vi "Generate.vi"(0 "reference in":refnum<class "Python.lvclass">, 1 "Path":path, 3 "Classes":T1[](array[typedef]), 5 "error in (no error)":errorcluster) -> (14 "reference out":refnum<class "Python.lvclass">, 19 "error out":errorcluster)   [LabVIEW 2018, in "Python.lvclass"]
uses:
  Python.lvclass
  Executer_class/typedefs/ClassDescription.ctl
  Executer_class/typedefs/MethodDescription.ctl
  Executer_class/Executer.lvclass
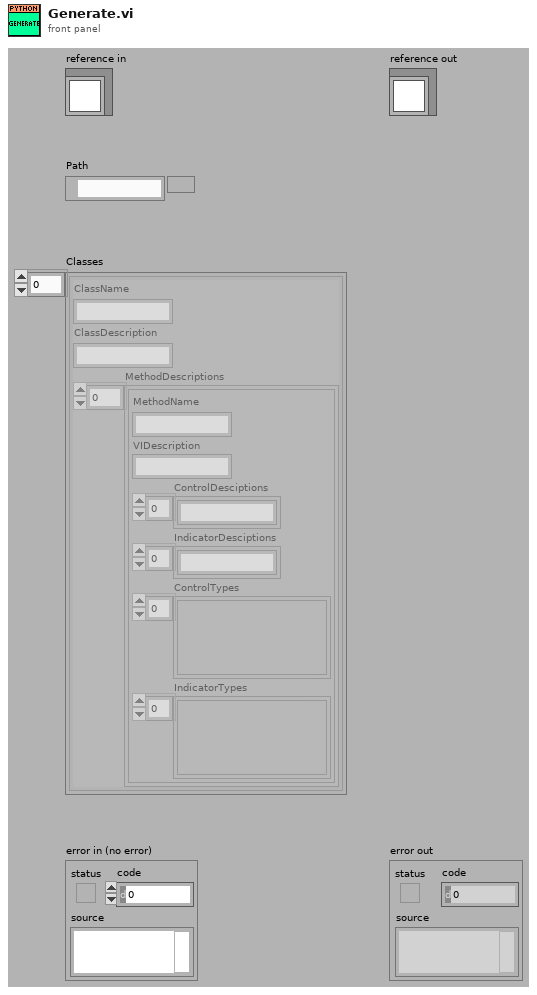
[diagram p1: front panel]
types:
  T1 = typedef "Executer.lvclass/ClassDescription.ctl" = cluster{"ClassName":string, "ClassDescription":string, "MethodDescriptions":T2[]}
  T2 = typedef "Executer.lvclass/MethodDescription.ctl" = cluster{"MethodName":string, "VIDescription":string, "ControlDesciptions":string[], "IndicatorDesciptions":string[], "ControlTypes":variant[], "IndicatorTypes":variant[]}
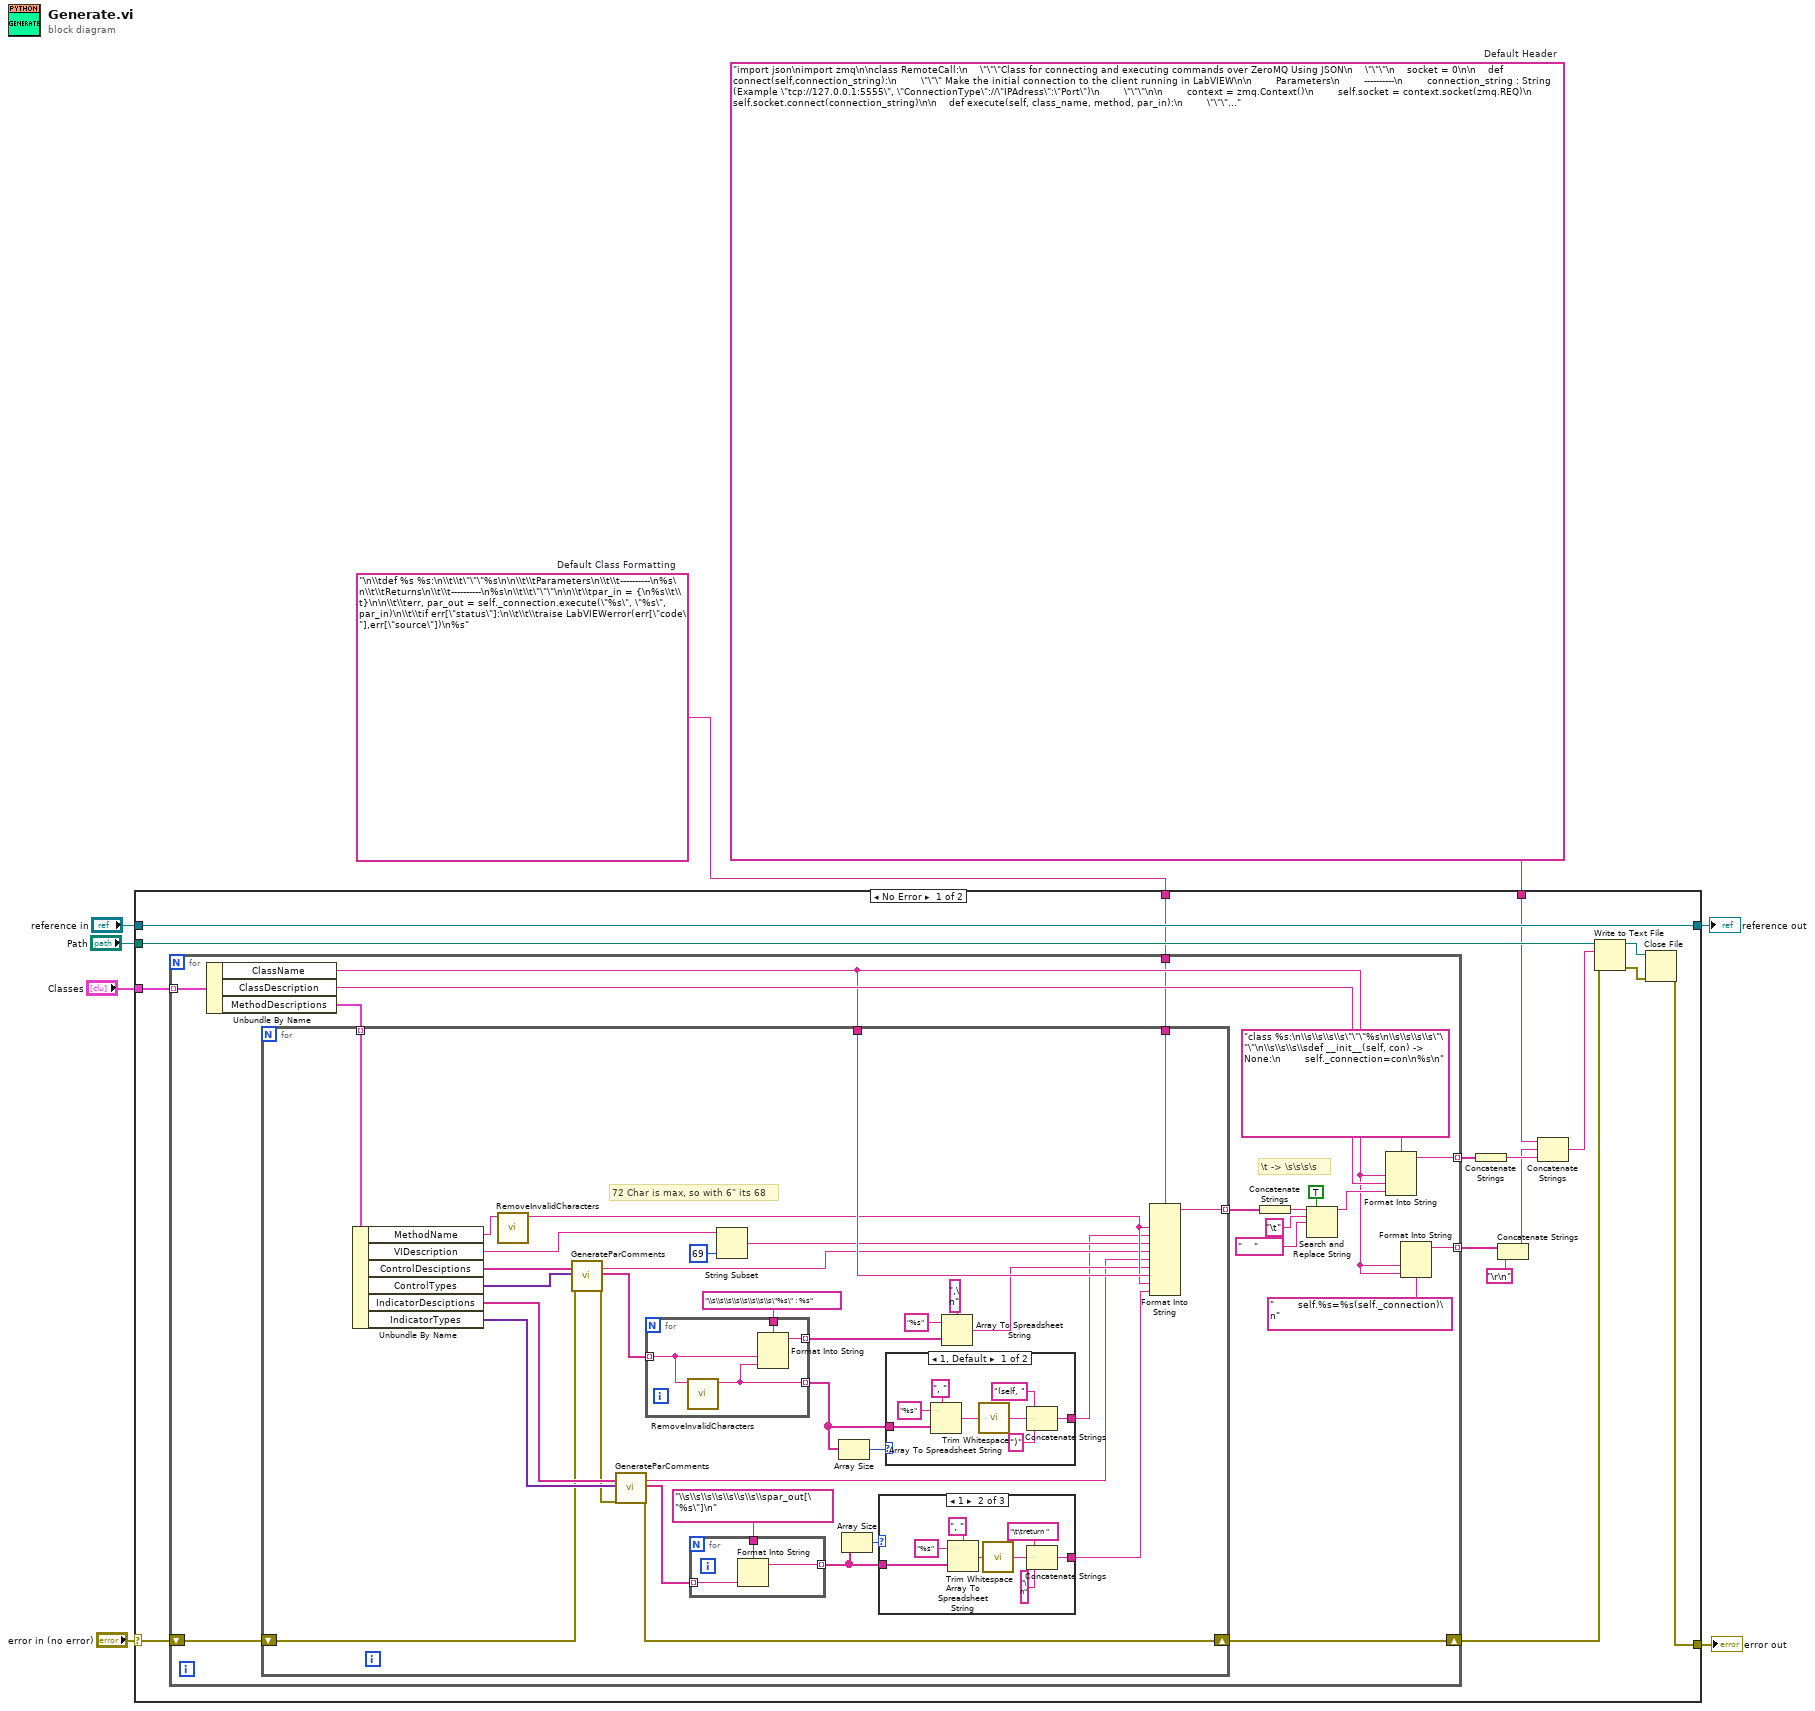
[diagram p0: block diagram]
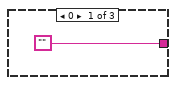
[diagram p2: hidden frame]
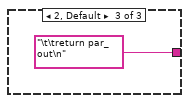
[diagram p3: hidden frame]
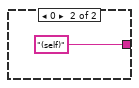
[diagram p4: hidden frame]
diagram:
  w1 = "\n\\tdef %s %s:\n\\t\\t\"\"\"%s\n\n\\t\\tParameters\n\\t\\t----------\n%s\n\\t\\tReturns\n\\t\\t----------\n%s\n\\t\\t\"\"\"\n\n\\t\\tpar_in = {\n%s\\t\\t}\n\n\\t\\terr, par_out = self._connection.execute(\"%s\", \"%s\", par_in)\n\\t\\tif err[\"status\"]:\n\\t\\t\\traise LabVIEWerror(err[\"code\"],err[\"source\"])\n%s"  # Default Class Formatting
  w2 = "import json\nimport zmq\n\nclass RemoteCall:\n    \"\"\"Class for connecting and executing commands over ZeroMQ Using JSON\n    \"\"\"\n    socket = 0\n\n    def connect(self,connection_string):\n        \"\"\" Make the initial connection to the client running in LabVIEW\n\n        Parameters\n        ----------\n        connection_string : String (Example \"tcp://127.0.0.1:5555\", \"ConnectionType\"://\"IPAdress\":\"Port\")\n        \"\"\"\n\n        context = zmq.Context()\n        self.socket = context.socket(zmq.REQ)\n        self.socket.connect(connection_string)\n\n    def execute(self, class_name, method, par_in):\n        \"\"\" Execute the Method by serializing inputs sending it over, and deserializing the result\n        \"\"\"\n        data_2_send = \"{ \\\"Command\\\":\\\"Execute\\\" }\\x17{\\\"ClassLabel\\\":\\\"%s\\\",\\\"Method\\\":\\\"%s\\\"}\\x17%s\" % (class_name, method, json.dumps({\"In\": par_in}))\n        self.socket.send_string (data_2_send)\n        message = self.socket.recv()\n        parts = message.split(chr(0x17).encode())\n        return json.loads(parts[1]), json.loads(parts[0])\n\nclass LabVIEWerror(Exception):\n    \"\"\"Base class for all LabVIEW errors\n\n    Attributes\n    ----------\n    code: error code for testing which error happend\n    source: source of the error\n    \"\"\"\n    def __init__(self, *args: object) -> None:\n        self.code = self.args[0]\n        self.source = self.args[1]\n        super().__init__(*args)\n\n    def __str__(self) -> str:\n        return f\"LabVIEW Error with code: {self.code} source: {self.source}\"\n\nclass LabviewControl:\n    \"\"\" Class for calling all labview function with connection embedded\n    \"\"\"\n\n    def __init__(self,connection_string) -> None:\n        self._connection=RemoteCall()\n        self._connection.connect(connection_string)\n"  # Default Header
  n1 = case shown="No Error" "error in (no error)" {
    selector: "error in (no error)" -> [w16 w101]
    tunnel: [w19 w101] -> w7
    tunnel: [w17 w100] -> w5
    tunnel: "reference in" -> [w17 w100]
    tunnel: "Classes" -> [w15 _]
    tunnel: "Path" -> [w14 _]
    tunnel: w2 -> [w12 _]
    tunnel: w1 -> [w9 _]
    frame No Error {
      n2 = for {
        tunnel: [w41] -> w24 mode=indexing
        tunnel: w15 -> [w31] mode=indexing
        shift-right: [w33] -> w18
        shift-left: w16 -> [w32]
        tunnel: [w26] -> w13 mode=indexing
        tunnel: w9 -> [w25]
        # "\\t -> \\s\\s\\s\\s"
        n3 = Unbundle By Name(w31) -> ("ClassName"=w27:string, "ClassDescription"=w30:string, "MethodDescriptions"=w29:T2[])
        n4 = for {
          tunnel: [w73] -> w40 mode=indexing
          tunnel: w27 -> [w72]
          shift-right: [w47] -> w33
          shift-left: w32 -> [w49]
          tunnel: w29 -> [w46] mode=indexing
          tunnel: w25 -> [w44]
          # "72 Char is max, so with 6\" its 68"
          n5 = Unbundle By Name(w46) -> ("MethodName"=w45:string, "VIDescription"=w61:string, "ControlDesciptions"=w60:string[], "ControlTypes"=w59:variant[], "IndicatorDesciptions"=w50:string[], "IndicatorTypes"=w51:variant[])
          n6 = call "RemoveInvalidCharacters.vi"("string in"=w45) -> ("string out"=w71:string)  [unwired: 10 in]
          n7 = call "GenerateParComments.vi"("Desciptions"=w60, "Types"=w59, "error in (no error)"=w49) -> ("DescriptionString"=w58:string, "Names"=w56:string[], "error out"=w48:errorcluster)  [unwired: 14 in]
          n8 = call "GenerateParComments.vi"("Desciptions"=w50, "Types"=w51, "error in (no error)"=w48) -> ("DescriptionString"=w57:string, "Names"=w55:string[], "error out"=w47:errorcluster)  [unwired: 14 in]
          n9 = for {
            tunnel: [w90] -> w65 mode=indexing
            tunnel: [w89] -> w53 mode=indexing
            tunnel: w56 -> [w88] mode=indexing
            tunnel: "\\s\\s\\s\\s\\s\\s\\s\\s\"%s\" : %s" ("string") -> [w87]
            n10 = call "RemoveInvalidCharacters.vi"("string in"=w88) -> ("string out"=w89:string)  [unwired: 10 in]
            n11 = Format Into String(format string=w87, w88, w89) -> (resulting string=w90:string)  [unwired: 2 in, 1 out]
          }
          n12 = for {
            tunnel: [w86] -> w66 mode=indexing
            tunnel: w55 -> [w85] mode=indexing
            tunnel: "\\s\\s\\s\\s\\s\\s\\s\\spar_out[\"%s\"]\n" ("string") -> [w84]
            n13 = Format Into String(format string=w84, w85) -> (resulting string=w86:string)  [unwired: 2 in, 1 out]
          }
          n14 = String Subset(string=w61, length (rest)=69 ("length (rest)")) -> (substring=w70:string)  [unwired: 1 in]
          n15 = Array Size(array=w53) -> (size(s)=w52:i32)
          n16 = Array Size(array=w66) -> (size(s)=w68:i32)
          n17 = case shown="1" w68 {
            tunnel: ["" w82 "\t\treturn par_out\n" ("string")] -> w67
            tunnel: w66 -> [_ w76 _]
            frame 0 {
            }
            frame 1 {
              n18 = Array To Spreadsheet String(delimiter (Tab)=", ", array=w76, 3:"%s" ("format string")) -> (spreadsheet string=w77:string)
              n19 = call <vilib>:"Trim Whitespace.vi"("string"=w77) -> ("trimmed string"=w75:string)  [unwired: 1 in]
              n20 = Concatenate Strings("\t\treturn " ("string"), w75, "\n" ("delimiter (Tab)")) -> (w82:string)
            }
            frame 2, Default {
            }
          }
          n21 = case shown="1, Default" w52 {
            tunnel: [w91 "(self)" ("string")] -> w54
            tunnel: w53 -> [w92 _]
            frame 1, Default {
              n22 = Array To Spreadsheet String(delimiter (Tab)=", ", array=w92, 3:"%s" ("format string")) -> (spreadsheet string=w95:string)
              n23 = call <vilib>:"Trim Whitespace.vi"("string"=w95) -> ("trimmed string"=w97:string)  [unwired: 1 in]
              n24 = Concatenate Strings("(self, " ("string"), w97, ")" ("string")) -> (w91:string)
            }
            frame 0 {
            }
          }
          n25 = Array To Spreadsheet String(delimiter (Tab)=",\n", array=w65, 3:"%s" ("format string")) -> (spreadsheet string=w62:string)
          n26 = Format Into String(format string=w44, w71, w54, w70, w58, w57, w62, w72, w71, w67) -> (resulting string=w73:string)  [unwired: 2 in, 1 out]
        }
        n27 = Concatenate Strings(w40) -> (w39:string)
        n28 = Search and Replace String(replace all?=TRUE ("replace all? (F)"), input string=w39, search string="\t", replace string="    " ("search string")) -> (result string=w34:string)  [unwired: 4 in, 3 out]
        n29 = Format Into String(format string="class %s:\n\\s\\s\\s\\s\"\"\"%s\n\\s\\s\\s\\s\"\"\"\n\\s\\s\\s\\sdef __init__(self, con) -> None:\n        self._connection=con\n%s\n", w27, w30, w34) -> (resulting string=w41:string)  [unwired: 2 in, 1 out]
        n30 = Format Into String(format string="        self.%s=%s(self._connection)\n", w27, w27) -> (resulting string=w26:string)  [unwired: 2 in, 1 out]
      }
      n31 = Concatenate Strings(w24) -> (w23:string)
      n32 = Concatenate Strings(w13, "\r\n") -> (w11:string)
      n33 = Concatenate Strings(w12, w11, w23) -> (w22:string)
      n34 = Write to Text File(file (use dialog)=w14, text=w22, error in=w18) -> (refnum out=w21:refnum<file>, error out=w20:errorcluster)  [unwired: 1 in, 1 out]
      n35 = Close File(refnum=w21, error in=w20) -> (error out=w19:errorcluster)  [unwired: 1 out]
    }
    frame Error {
    }
  }
  "error out" <- w7
  "reference out" <- w5
